vi "FT26_6 to SGL.vi"(1 "26.6":i32) -> (0 "sgl":sgl)   [LabVIEW 2023, in "Freetype Drawer.lvlib"]
uses:
  Freetype Drawer.lvlib
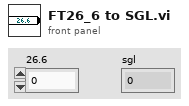
[diagram p1: front panel]
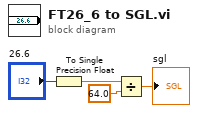
[diagram p0: block diagram]
diagram:
  n1 = To Single Precision Float(number="26.6") -> (single precision float=w1:sgl)
  n2 = Divide(x=w1, y=sgl 64.0) -> (x/y=→"sgl":sgl)
